vi "IBM4_Read(VN).vi"(8 "error in":errorcluster, 9 "Number":i32=10, 10 "Channel":i32=3 min=0 max=4, 11 "COM resource in":refnum<visa-resource-name>="ASRL5::INSTR") -> (0 "error out":errorcluster, 2 "array":dbl[](array[numeric]), 3 "COM resource out":refnum<visa-resource-name>="ASRL5::INSTR")   [LabVIEW 2022 SP3, in "IBM4.lvlib"]
doc: "This VI interfaces with the IBM4 to perform a read operation.\n\nThe input channel must be between 0 and 3, And the number of readings should be greater than zero. At some point the number of reading will be too high and will cause a timeout error. This should only happen for numbers larger than 10000. The output will be an array of floating point (Voltage) values.\n\nAlternate read operations exist covering binary or floating point, single reading, multiple readings, and an average of multiple readings (floating point only)."
uses:
  <instrlib>/IBM4/IBM4.lvlib
panel:
  out "read buffer":string="Output 3 = 1.85786 \r\n"
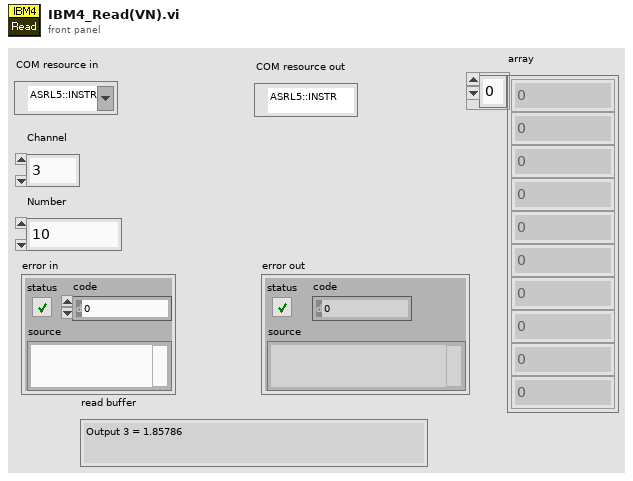
[diagram p1: front panel]
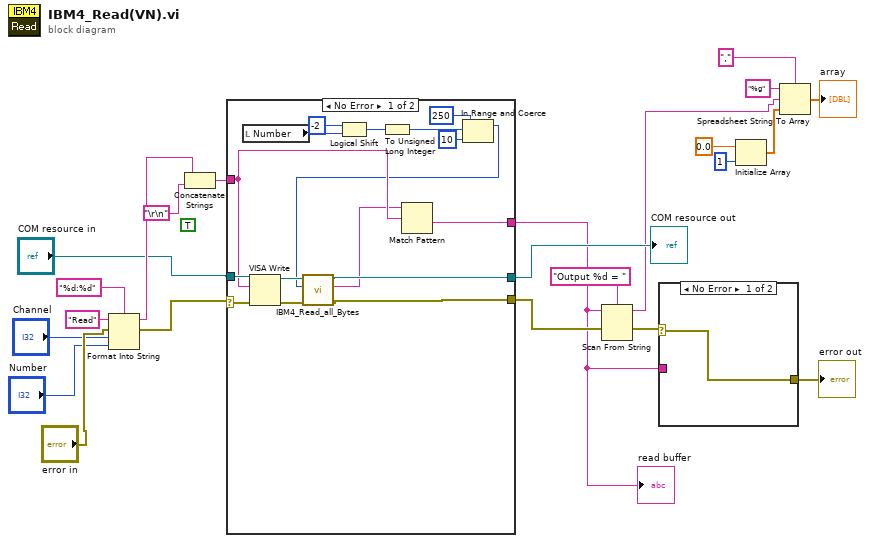
[diagram p0: block diagram]
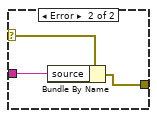
[diagram p2: hidden frame]
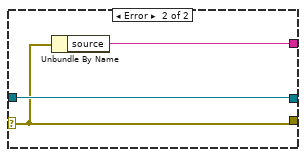
[diagram p3: hidden frame]
diagram:
  (unwired) TRUE ("Enable Termination\nChar (T)")
  n1 = Format Into String(format string="%d:%d", initial string="Read", error in="error in", "Channel", "Number") -> (resulting string=w14:string, error out=w1:errorcluster)
  n2 = Concatenate Strings(w14, "\r\n") -> (w13:string)
  n3 = case shown="No Error" w1 {
    selector: w1 -> [w36 w41]
    tunnel: "COM resource in" -> [w39 w42]
    tunnel: [w25 w41] -> w17
    tunnel: [w38 w40] -> w10
    tunnel: w13 -> [w37 _]
    tunnel: [w26 w42] -> w18
    frame No Error {
      n4 = local read "Number"() -> (w32:i32)
      n5 = VISA Write(VISA resource name=w39, write buffer=w37, error in (no error)=w36) -> (VISA resource name out=w29:refnum<visa-resource-name>, error out=w28:errorcluster)  [unwired: 1 out]
      n6 = Logical Shift(y=i16 -2, x=w32) -> (x << y=w33:i32)
      n7 = To Unsigned Long Integer(number=w33) -> (unsigned 32bit integer=w30:u32)
      n8 = In Range and Coerce(upper limit=u32 250, x=w30, lower limit=u32 10) -> (coerced(x)=w27:u32)  [unwired: 1 out]
      n9 = call <instrlib>:"IBM4_Read_all_Bytes.vi"("error in (no error)"=w28, "milliseconds to wait"=w27, "VISA Refnum in"=w29) -> ("error out"=w25:errorcluster, "String"=w24:string, "VISA Refnum out"=w26:refnum<visa-resource-name>)  [unwired: 2 in]
      n10 = Match Pattern(string=w24, regular expression=w37) -> (after substring=w38:string)  [unwired: 1 in, 3 out]
    }
    frame Error {
      n11 = Unbundle By Name(w41) -> ("source"=w40:string)
    }
  }
  "COM resource out" <- w18
  "read buffer" <- w10
  n12 = Scan From String(format string="Output %d = ", input string=w10, error in=w17) -> (remaining string=w4:string, error out=w12:errorcluster)  [unwired: 3 in, 1 out]
  n13 = case shown="No Error" w12 {
    selector: w12 -> [w43 w46]
    tunnel: [w43 w44] -> w11
    tunnel: w10 -> [_ w45]
    frame No Error {
    }
    frame Error {
      n14 = Bundle By Name(cluster=w46, "source"=w45) -> (w44:errorcluster)
    }
  }
  "error out" <- w11
  n15 = Initialize Array(0.0, 1 ("dimension size")) -> (w8:dbl[])
  n16 = Spreadsheet String To Array(delimiter (Tab)=",", format string="%g", spreadsheet string=w4, array type (2D Dbl)=w8) -> (array=→"array":dbl[])
